vi "run_autoWC_v0.007.vi"(7 "long?":bool=TRUE, 8 "error in":errorcluster, 9 "HEK/slice options":enum16{"slice", "HEK"}(ring), 10 "auto run?":bool=TRUE, 11 "data in":T3={"daq_ao 1"="Dev1/ao0", "daq_ai 1"="Dev1/ai0", "experiment day folder"=path "C:/Users/sftlab/Documents/patcherBot_exp/data/test.lvm", "Multiclamp init error"=0, "Multiclamp Handle Out"=0, "sampling rate (Hz)"=20000, "trial name"=""}) -> (0 "error out":errorcluster)   [LabVIEW 2015]
uses:
  controls/Load and Save Controls_LV2009.llb/RWC_Actions.ctl
  wc_protocol_v1.003 Folder/whole_cell_protocol/Controls/clamp_profile.ctl
  controls/memtest_def.ctl
  Controls/Data.ctl
  wc_protocol_v1.003 Folder/whole_cell_protocol/Controls/cell_stats-v02.ctl
panel:
  out "HEK/slice options string":string
  out "config file":path=path "C:/multiBot/patcherBot/autoWCconfigs/autoWC_config_neuron-v07.ini"
  in  "load":bool
  in  "texts":enum32{"status", "comments", "release notes"}(tab)
  out "status":string
  in  "trial comments":string
  in  "release notes":string
  out "cell stats":T1 {"STD" format="%010.2f"; "Variance" format="%010.2f"; "Rt (MOhms)" format="%010.2f"; "tau (ms)" format="%08.2g"; "Cm (pF)" format="%08.2f"; "Ra (MOhms)" format="%010.2f"; "Rm (MOhms)" format="%010.2f"; "Ihold (pA)" format="%010.2f"}
  in  "save":bool
  in  "stop":bool
  in  "output":enum32{"VClamp", "IClamp"}(tab)
  out "Recorded currents (pA)":waveform(dbl)[](graph)
  out "Command steps (mV)":waveform(dbl)[](graph)
  out "Command steps (pA)":waveform(dbl)[](graph)
  out "Recorded voltage (mV)":waveform(dbl)[](graph)
  in  "run":bool
  in  "save as...":bool
  in  "update plots":bool
  in  "protocol creation":T2(tab)
  in  "DEBUG?":bool
  in  "auto WC run trigger":bool
  in  "twitter?":bool
  in  "config for long protocol":path=path "C:/multiBot/patcherBot/autoWCconfigs/autoWC_config_cellAttached-v01.ini"
  in  "config for standard protocol":path=path "C:/multiBot/patcherBot/autoWCconfigs/autoWC_config_neuron-v07.ini"
  in  "starting set":enum32{"Iprot", "Vprot", "Imemtest", "Vmemtest"}(tab)
  out "starting iprot cmd":waveform(dbl)[](graph)
  in  "Starting Iprot":T5={"Iclamp in"={"aLevel"=0.0, "aDelta"=0.0, "aDuration"=4000, "bLevel"=-200.0, "bDelta"=100.0, "bDuration"=4000, "cLevel"=0.0, "cDelta"=0.0, "cDuration"=4000}, "# iter"=6, "# reps IC"=1}
  out "starting vprot cmd":waveform(dbl)[](graph)
  in  "Starting Vprot":T6={"Vclamp in"={"aLevel"=0.0, "aDelta"=0.0, "aDuration"=40000, "bLevel"=-30.0, "bDelta"=10.0, "bDuration"=40000, "cLevel"=0.0, "cDelta"=0.0, "cDuration"=40000}, "# iter"=8, "# reps VC"=1}
  out "starting imemtest view":waveform(dbl)(graph)
  in  "Starting Iclamp memtest":T7={"Samples to Read"=2000, "Rate (Hz)"=20000.0, "Amplitude (mV/pA)"=-50.0, "Offset (mV/pA)"=0.0, "Frequency (Hz)"=10.0, "duty cycle (%)"=50.0, "phase"=0.0} {"phase" format="%.2p"; "duty cycle (%)" format="%0.2f"}
  out "starting vmemtest view":waveform(dbl)(graph)
  in  "Starting Vclamp memtest":T7={"Samples to Read"=2000, "Rate (Hz)"=20000.0, "Amplitude (mV/pA)"=10.0, "Offset (mV/pA)"=0.0, "Frequency (Hz)"=10.0, "duty cycle (%)"=50.0, "phase"=-90.0} {"phase" format="%.2p"; "duty cycle (%)" format="%0.2f"}
  in  "wait after init (s)":dbl
  in  "Starting sets":T8
  in  "wait after Starting set (s)":dbl
  in  "wait after Repeating set (s)":dbl
  in  "# sets":i32=18
  in  "Repeating sets":T8
  in  "repeating set":enum32{"Iprot", "Vprot", "Imemtest", "Vmemtest"}(tab)
  out "repeating iprot cmd":waveform(dbl)[](graph)
  in  "Repeating Iprot":T5={"Iclamp in"={"aLevel"=0.0, "aDelta"=0.0, "aDuration"=4000, "bLevel"=-200.0, "bDelta"=100.0, "bDuration"=4000, "cLevel"=0.0, "cDelta"=0.0, "cDuration"=4000}, "# iter"=6, "# reps IC"=1}
  out "repeating vprot cmd":waveform(dbl)[](graph)
  in  "Repeating Vprot":T6={"Vclamp in"={"aLevel"=0.0, "aDelta"=0.0, "aDuration"=40000, "bLevel"=-30.0, "bDelta"=10.0, "bDuration"=40000, "cLevel"=0.0, "cDelta"=0.0, "cDuration"=40000}, "# iter"=8, "# reps VC"=1}
  out "repeating imemtest cmd":waveform(dbl)(graph)
  in  "Repeating Iclamp memtest":T7={"Samples to Read"=2000, "Rate (Hz)"=20000.0, "Amplitude (mV/pA)"=-50.0, "Offset (mV/pA)"=0.0, "Frequency (Hz)"=10.0, "duty cycle (%)"=50.0, "phase"=0.0} {"phase" format="%.2p"; "duty cycle (%)" format="%0.2f"}
  out "repeating vmemtest cmd":waveform(dbl)(graph)
  in  "Repeating Vclamp memtest":T7={"Samples to Read"=2000, "Rate (Hz)"=20000.0, "Amplitude (mV/pA)"=10.0, "Offset (mV/pA)"=0.0, "Frequency (Hz)"=10.0, "duty cycle (%)"=50.0, "phase"=-90.0} {"phase" format="%.2p"; "duty cycle (%)" format="%0.2f"}
  in  "wait between protocols (s)":dbl
  in  "wait between sets (s)":dbl
  in  "ending set":enum32{"Iprot", "Vprot", "Imemtest", "Vmemtest"}(tab)
  out "ending iprot cmd":waveform(dbl)[](graph)
  in  "Ending Iprot":T5={"Iclamp in"={"aLevel"=0.0, "aDelta"=0.0, "aDuration"=4000, "bLevel"=-200.0, "bDelta"=100.0, "bDuration"=4000, "cLevel"=0.0, "cDelta"=0.0, "cDuration"=4000}, "# iter"=6, "# reps IC"=1}
  out "ending vprot cmd":waveform(dbl)[](graph)
  in  "Ending Vprot":T6={"Vclamp in"={"aLevel"=0.0, "aDelta"=0.0, "aDuration"=40000, "bLevel"=-30.0, "bDelta"=10.0, "bDuration"=40000, "cLevel"=0.0, "cDelta"=0.0, "cDuration"=40000}, "# iter"=8, "# reps VC"=1}
  out "ending imemtest cmd":waveform(dbl)(graph)
  in  "Ending Iclamp memtest":T7={"Samples to Read"=2000, "Rate (Hz)"=20000.0, "Amplitude (mV/pA)"=-50.0, "Offset (mV/pA)"=0.0, "Frequency (Hz)"=10.0, "duty cycle (%)"=50.0, "phase"=0.0} {"phase" format="%.2p"; "duty cycle (%)" format="%0.2f"}
  out "ending vmemtest cmd":waveform(dbl)(graph)
  in  "Ending Vclamp memtest":T7={"Samples to Read"=2000, "Rate (Hz)"=20000.0, "Amplitude (mV/pA)"=10.0, "Offset (mV/pA)"=0.0, "Frequency (Hz)"=10.0, "duty cycle (%)"=50.0, "phase"=-90.0} {"phase" format="%.2p"; "duty cycle (%)" format="%0.2f"}
  in  "Ending sets":T8
  in  "holding memtest":bool
  in  "holding set":enum32{"VClamp", "IClamp"}(tab)
  out "holding vmemtest cmd":waveform(dbl)(graph)
  in  "holding Vclamp memtest":T7={"Samples to Read"=2000, "Rate (Hz)"=20000.0, "Amplitude (mV/pA)"=10.0, "Offset (mV/pA)"=0.0, "Frequency (Hz)"=10.0, "duty cycle (%)"=50.0, "phase"=0.0} {"phase" format="%.2p"; "duty cycle (%)" format="%0.2f"}
  out "holding imemtest cmd":waveform(dbl)(graph)
  in  "holding Iclamp memtest":T7={"Samples to Read"=2000, "Rate (Hz)"=20000.0, "Amplitude (mV/pA)"=-50.0, "Offset (mV/pA)"=0.0, "Frequency (Hz)"=10.0, "duty cycle (%)"=50.0, "phase"=0.0} {"phase" format="%.2p"; "duty cycle (%)" format="%0.2f"}
  # "IClamp step protocol"
  # "x"
  # "VClamp step protocol"
  # "x"
  # "IClamp step protocol"
  # "x"
  # "VClamp step protocol"
  # "x"
  # "IClamp step protocol"
  # "x"
  # "VClamp step protocol"
  # "x"
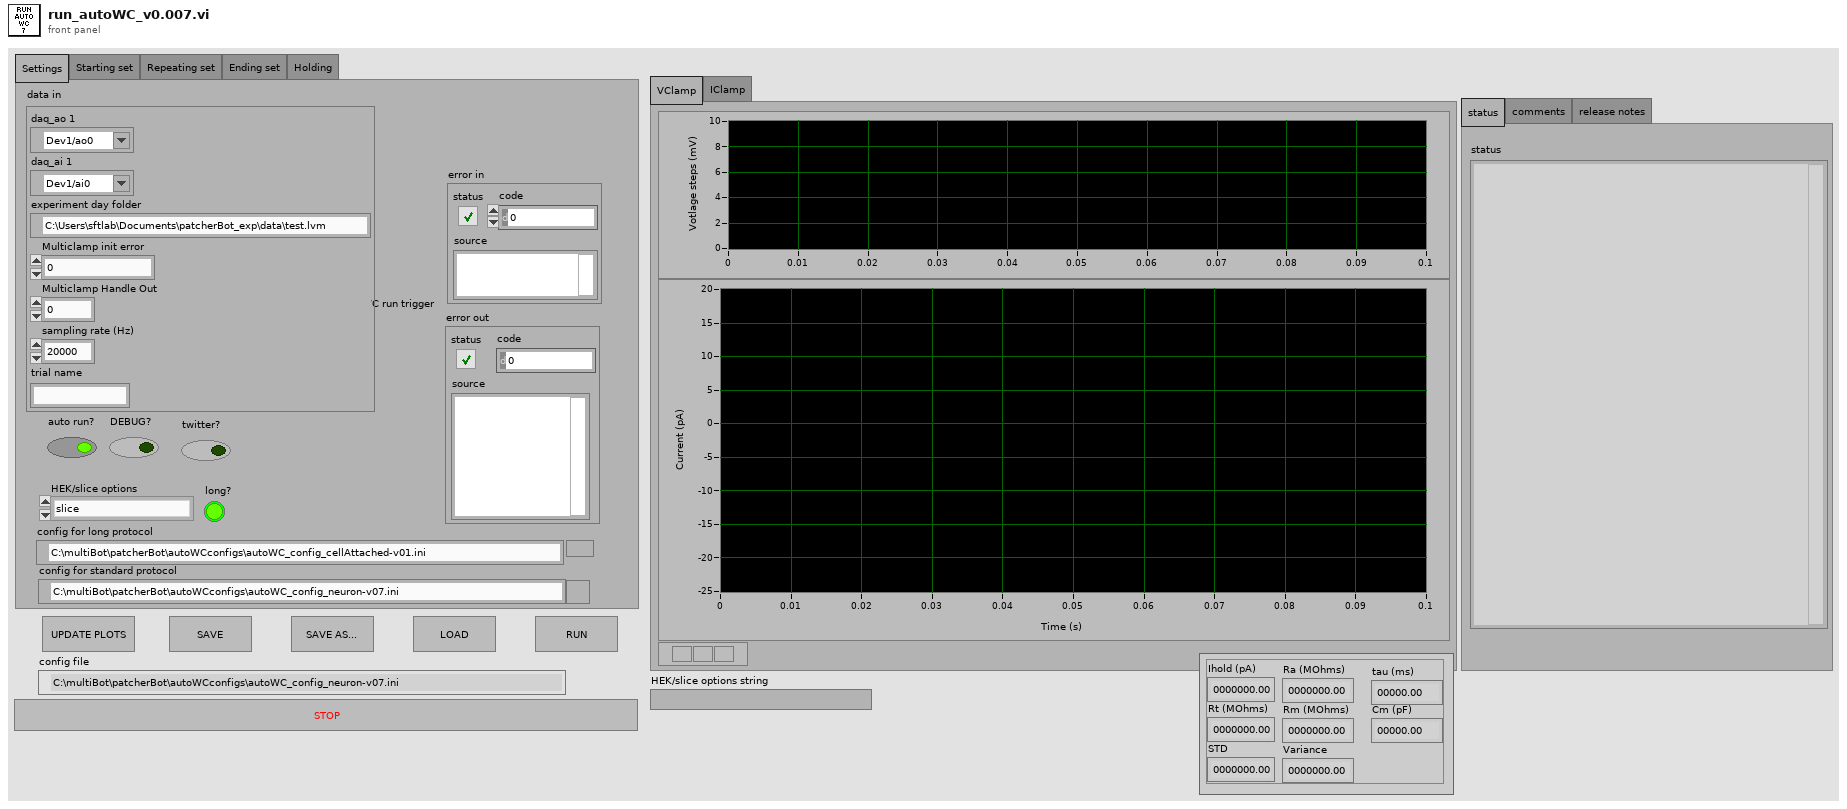
[diagram p1: front panel]
types:
  T1 = typedef "cell_stats-v02.ctl" = cluster{"Ihold (pA)":dbl, "Rm (MOhms)":dbl, "Ra (MOhms)":dbl, "Cm (pF)":dbl, "tau (ms)":dbl, "Rt (MOhms)":dbl, "Variance":dbl, "STD":dbl}
  T2 = enum32{"Settings", "Starting set", "Repeating set", "Ending set", "Holding"}
  T3 = typedef "Data.ctl" = cluster{"daq_ao 1":tag, "daq_ai 1":tag, "experiment day folder":path, "Multiclamp init error":i32, "Multiclamp Handle Out":u32, "sampling rate (Hz)":i32, "trial name":string}
  T4 = typedef "clamp_profile.ctl" = cluster{"aLevel":dbl, "aDelta":dbl, "aDuration":i32, "bLevel":dbl, "bDelta":dbl, "bDuration":i32, "cLevel":dbl, "cDelta":dbl, "cDuration":i32}
  T5 = cluster{"Iclamp in":T4, "# iter":i32, "# reps IC":i32}
  T6 = cluster{"Vclamp in":T4, "# iter":i32, "# reps VC":i32}
  T7 = typedef "memtest_def.ctl" = cluster{"Samples to Read":i32, "Rate (Hz)":dbl, "Amplitude (mV/pA)":dbl, "Offset (mV/pA)":dbl, "Frequency (Hz)":dbl, "duty cycle (%)":dbl, "phase":dbl}
  T8 = cluster{" Iprot":bool, " Vprot":bool, " Imemtest":bool, " Vmemtest":bool}
  T9 = typedef "RWC_Actions.ctl" = enum16{"Read", "Write", "Read and Create"}
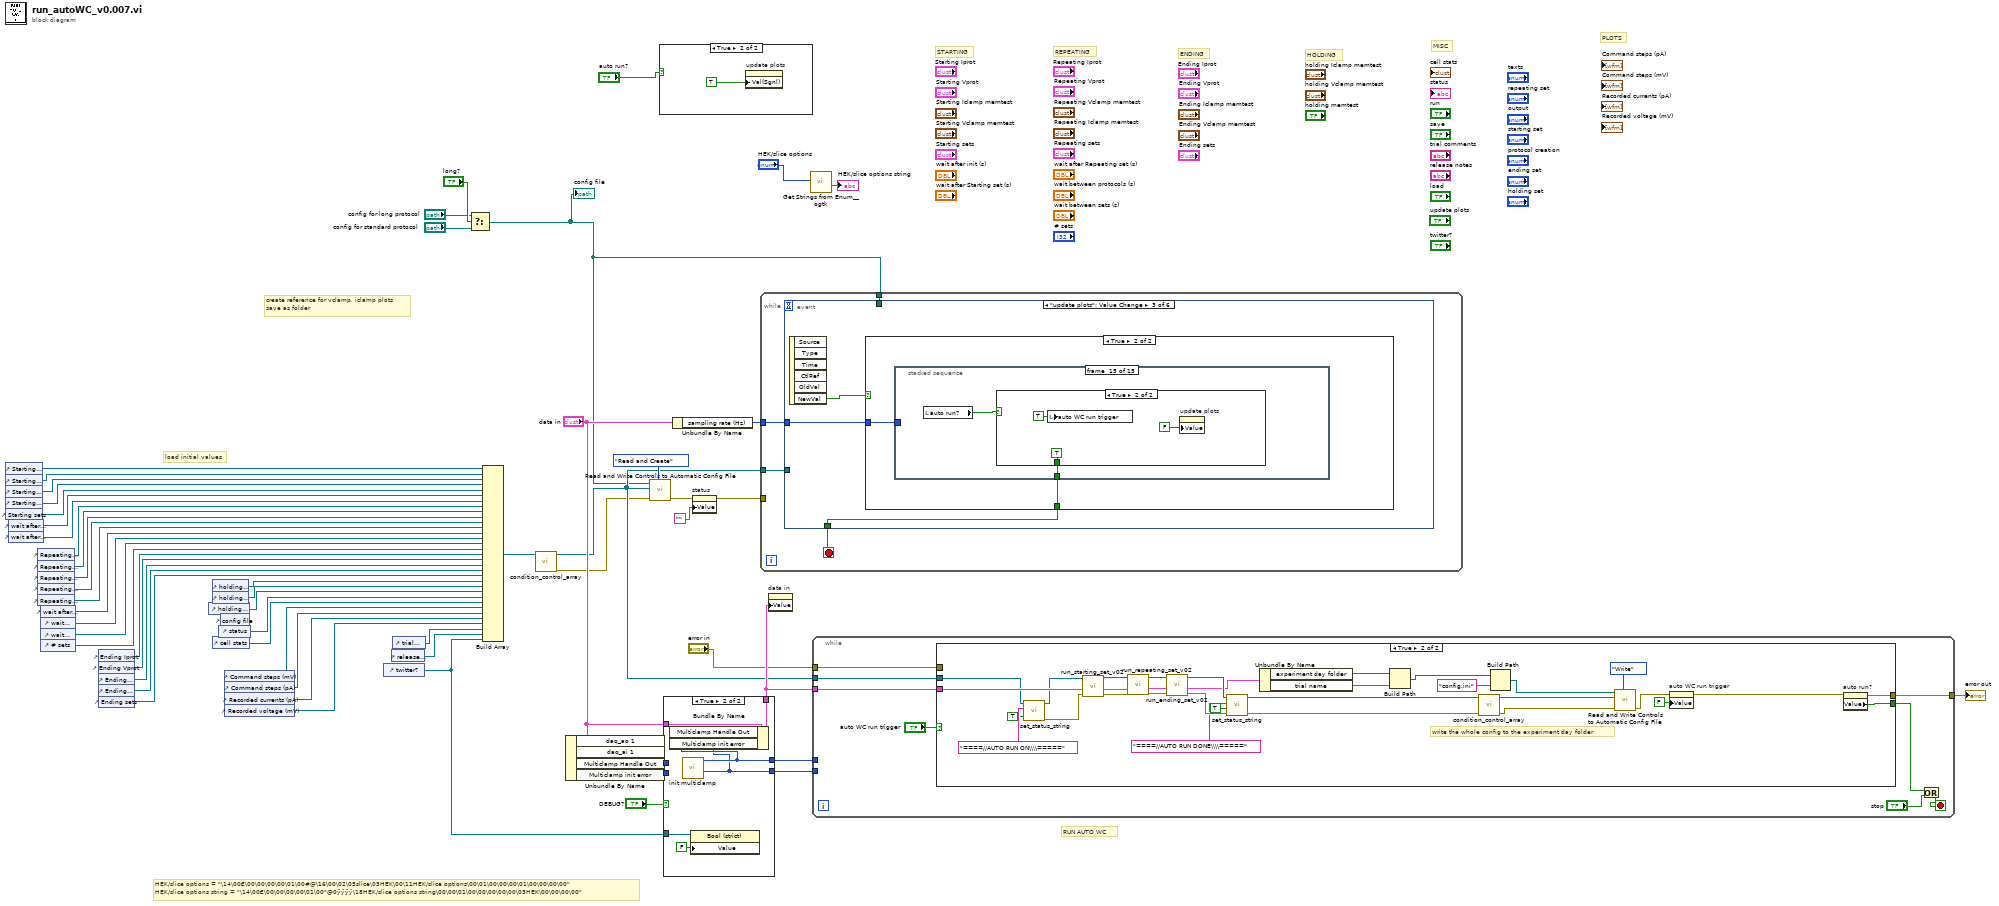
[diagram p0: block diagram]
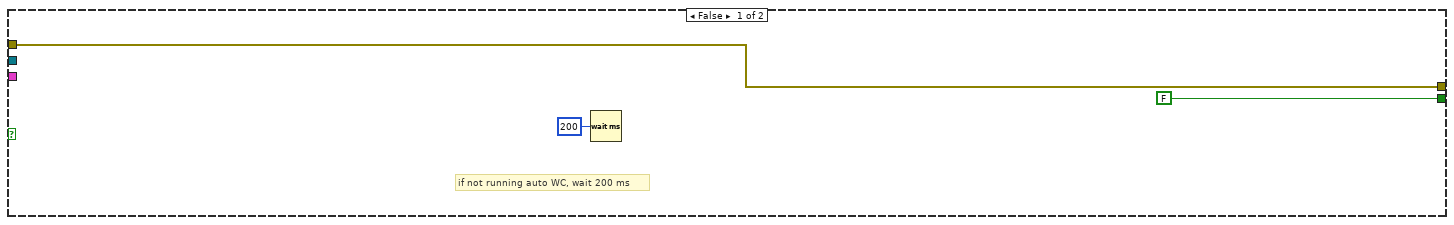
[diagram p4: hidden frame]
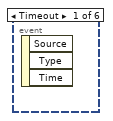
[diagram p5: hidden frame]
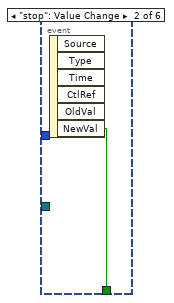
[diagram p6: hidden frame]
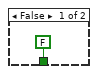
[diagram p7: hidden frame]
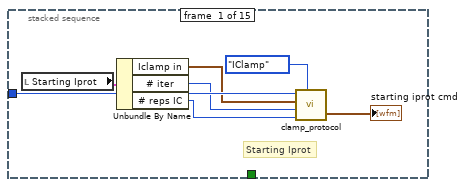
[diagram p8: hidden frame]
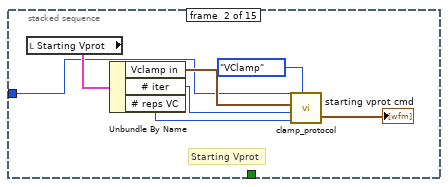
[diagram p9: hidden frame]
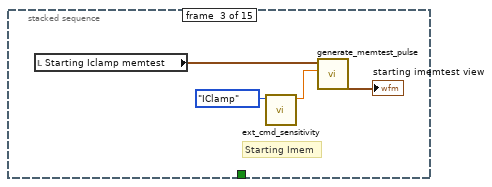
[diagram p10: hidden frame]
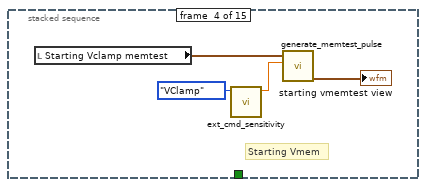
[diagram p11: hidden frame]
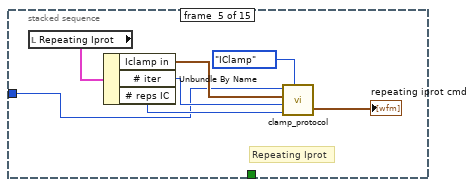
[diagram p12: hidden frame]
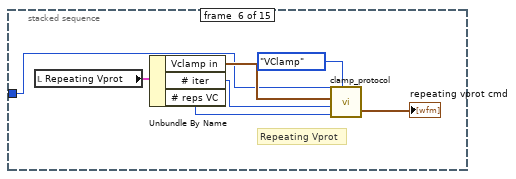
[diagram p13: hidden frame]
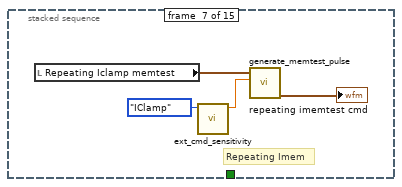
[diagram p14: hidden frame]
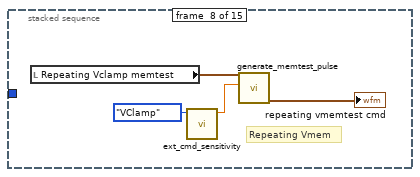
[diagram p15: hidden frame]
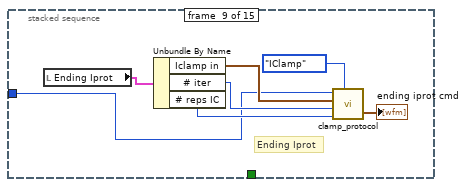
[diagram p16: hidden frame]
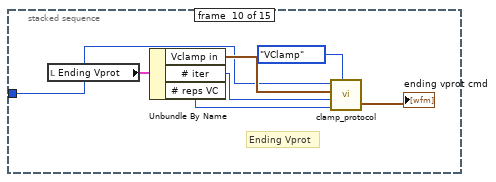
[diagram p17: hidden frame]
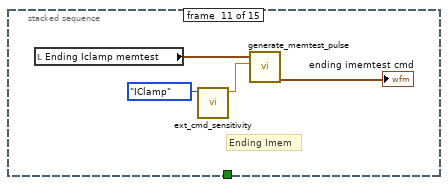
[diagram p18: hidden frame]
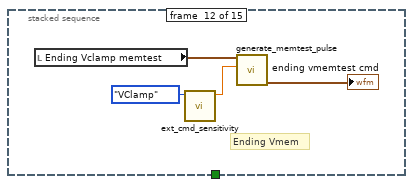
[diagram p19: hidden frame]
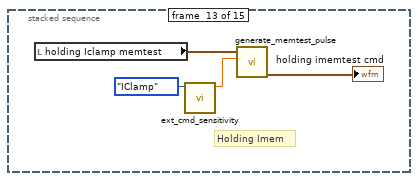
[diagram p20: hidden frame]
diagram:
  # "HEK/slice options = \"\\14\\00€\\00\\00\\00\\00\\01\\00#@\\16\\00\\02\\05slice\\03HEK\\00\\11HEK/slice options\\00\\01\\00\\00\\00\\01\\00\\00\\00\\00\"\nHEK/slice options string = \"\\14\\00€\\00\\00\\00\\00\\01\\00\"@0ÿÿÿÿ\\18HEK/slice options string\\00\\00\\01\\00\\00\\00\\00\\00\\03HEK\\00\\00\\00\\00\""
  # "PLOTS"
  # "MISC"
  # "create reference for vclamp, iclamp plots\nsave as folder"
  # "load initial values"
  # "HOLDING"
  # "ENDING"
  # "REPEATING"
  # "STARTING"
  # "RUN AUTO WC"
  n1 = control-ref of="Starting Iprot"() -> (w35:refnum<vi>)
  n2 = control-ref of="Starting Vprot"() -> (w34:refnum<vi>)
  n3 = control-ref of="Starting Iclamp memtest"() -> (w33:refnum<vi>)
  n4 = control-ref of="Starting Vclamp memtest"() -> (w32:refnum<vi>)
  n5 = control-ref of="Starting sets"() -> (w36:refnum<vi>)
  n6 = control-ref of="wait after init (s)"() -> (w37:refnum<vi>)
  n7 = control-ref of="wait after Starting set (s)"() -> (w38:refnum<vi>)
  n8 = control-ref of="Repeating Iprot"() -> (w39:refnum<vi>)
  n9 = control-ref of="Repeating Vprot"() -> (w40:refnum<vi>)
  n10 = control-ref of="Repeating Vclamp memtest"() -> (w41:refnum<vi>)
  n11 = control-ref of="Repeating Iclamp memtest"() -> (w42:refnum<vi>)
  n12 = control-ref of="Repeating sets"() -> (w43:refnum<vi>)
  n13 = control-ref of="wait after Repeating set (s)"() -> (w44:refnum<vi>)
  n14 = control-ref of="wait between protocols (s)"() -> (w45:refnum<vi>)
  n15 = control-ref of="wait between sets (s)"() -> (w46:refnum<vi>)
  n16 = control-ref of="# sets"() -> (w47:refnum<vi>)
  n17 = control-ref of="Ending Iprot"() -> (w48:refnum<vi>)
  n18 = control-ref of="Ending Vprot"() -> (w49:refnum<vi>)
  n19 = control-ref of="Ending Iclamp memtest"() -> (w50:refnum<vi>)
  n20 = control-ref of="Ending Vclamp memtest"() -> (w51:refnum<vi>)
  n21 = control-ref of="Ending sets"() -> (w52:refnum<vi>)
  n22 = control-ref of="holding memtest"() -> (w55:refnum<vi>)
  n23 = control-ref of="holding Iclamp memtest"() -> (w53:refnum<vi>)
  n24 = control-ref of="holding Vclamp memtest"() -> (w54:refnum<vi>)
  n25 = control-ref of="cell stats"() -> (w26:refnum<vi>)
  n26 = control-ref of="status"() -> (w27:refnum<vi>)
  n27 = control-ref of="config file"() -> ()  [unwired: 1 out]
  n28 = control-ref of="Command steps (mV)"() -> (w14:refnum<vi>)
  n29 = control-ref of="Command steps (pA)"() -> (w13:refnum<vi>)
  n30 = control-ref of="Recorded currents (pA)"() -> (w12:refnum<vi>)
  n31 = control-ref of="Recorded voltage (mV)"() -> (w11:refnum<vi>)
  n32 = control-ref of="twitter?"() -> (w7:refnum<vi>)
  n33 = control-ref of="release notes"() -> (w15:refnum<vi>)
  n34 = control-ref of="trial comments"() -> (w16:refnum<vi>)
  n35 = Select(t="config for long protocol", s="long?", f="config for standard protocol") -> (s? t:f=w1:path)
  "config file" <- w1
  n36 = Build Array(w35, w34, w33, w32, w36, w37, w38, w39, w40, w41, w42, w43, w44, w45, w46, w47, w48, w49, w50, w51, w52, w53, w54, w55, w27, w26, w14, w13, w12, w11, w16, w15, w7) -> (w10:refnum<vi>[])
  n37 = call "condition_control_array.vi"("control array in"=w10) -> ("error out"=w8:errorcluster, "control array out"=w9:refnum<vi>[])  [unwired: 9 in]
  n38 = Unbundle By Name("data in") -> ("Multiclamp Handle Out"=w25:u32, "Multiclamp init error"=w24:i32)  [unwired: 2 out]
  n39 = call "Read and Write Controls to Automatic Config File.vi"("Action"=RWC_Actions."Read and Create", "error in"=w8, "Control References"=w9, "filepath"=w1) -> ("error out"=w23:errorcluster)  [unwired: 7 in]
  n40 = case shown="True" "auto run?" {
    frame False {
    }
    frame True {
      n41 = property on="update plots" class="Bool (strict)"("Val(Sgnl)"=TRUE ("update plots")) -> ()  [unwired: 2 in, 2 out]
    }
  }
  n42 = case shown="True" "DEBUG?" {
    tunnel: [w61 w67] -> w29
    tunnel: [w60 w66] -> w28
    tunnel: w25 -> [w61 _]
    tunnel: w24 -> [w60 _]
    tunnel: "data in" -> [w59 w65]
    tunnel: [w59 w64] -> w19
    tunnel: w7 -> [_ w63]
    frame False {
    }
    frame True {
      n43 = call "init multiclamp.vi"() -> ("Error out"=w66:i32, "Multiclamp Handle Out"=w67:u32)  [unwired: 9 in, 1 out]
      n44 = Bundle By Name(cluster=w65, "Multiclamp Handle Out"=w67, "Multiclamp init error"=w66) -> (w64:T3)
      n45 = property class="Bool (strict)"(reference=w63, "Value"=FALSE) -> ()  [unwired: 1 in, 2 out]
    }
  }
  n46 = Unbundle By Name("data in") -> ("sampling rate (Hz)"=w56:i32)
  n47 = property on="status" class="Str"(error in=w23, "Value"="") -> (error out=w22:errorcluster)  [unwired: 1 in, 1 out]
  n48 = while {
    tunnel: w56 -> [w70]
    tunnel: w1 -> [w69]
    tunnel: w22 -> [_]
    tunnel: w9 -> [w68]
    stop <- w71 stop-if-true
    n49 = event shown="[2] \"update plots\": Value Change" {
      selector: _ -> [_ _ _ _ _ _]
      dyn-events: _ -> [_ _ _ _ _ _]
      timeout: _ -> [_ _ _ _ _ _]
      tunnel: [_ w72 w73 _ _ _] -> w71
      tunnel: w70 -> [_ _ w74 _ _ _]
      tunnel: w69 -> [_ _ _ _ w163 _]
      tunnel: w68 -> [_ _ _ _ w162 w179]
      event Timeout {
        n50 = event-data() -> ()  [unwired: 1 in, 3 out]
      }
      event "stop": Value Change {
        n51 = event-data() -> ("NewVal"=w72:bool)  [unwired: 1 in, 5 out]
      }
      event "update plots": Value Change {
        n52 = event-data() -> ("NewVal"=w75:bool)  [unwired: 1 in, 5 out]
        n53 = case shown="True" w75 {
          tunnel: w74 -> [_ w78]
          tunnel: [FALSE w77] -> w73
          frame False {
          }
          frame True {
            n54 = stacked-sequence {
              tunnel: w78 -> [w85 w86 _ _ w103 w109 _ _ w123 w131 _ _ _ _ _]
              tunnel: [_ _ _ _ _ _ _ _ _ _ _ _ _ _ w153] -> w77
              frame #0 {
                # "Starting Iprot"
                n55 = local read "Starting Iprot"() -> (w83:T5)
                n56 = Unbundle By Name(w83) -> ("Iclamp in"=w82:T4, "# iter"=w81:i32, "# reps IC"=w80:i32)
                n57 = call "clamp_protocol.vi"("which clamp"=enum16{"VClamp", "IClamp"}."IClamp", "# reps"=w80, "# Iterations"=w81, "clamp in"=w82, "sampling rate (Hz)"=w85) -> ("View profile (wvfrms)"=→"starting iprot cmd":waveform(dbl)[])  [unwired: 2 out]
              }
              frame #1 {
                # "Starting Vprot"
                n58 = local read "Starting Vprot"() -> (w90:T6)
                n59 = Unbundle By Name(w90) -> ("Vclamp in"=w91:T4, "# iter"=w88:i32, "# reps VC"=w87:i32)
                n60 = call "clamp_protocol.vi"("which clamp"=enum16{"VClamp", "IClamp"}."VClamp", "# reps"=w87, "# Iterations"=w88, "clamp in"=w91, "sampling rate (Hz)"=w86) -> ("View profile (wvfrms)"=→"starting vprot cmd":waveform(dbl)[])  [unwired: 2 out]
              }
              frame #2 {
                # "Starting Imem"
                n61 = local read "Starting Iclamp memtest"() -> (w93:T7)
                n62 = call "ext_cmd_sensitivity.vi"("which clamp"=enum16{"VClamp", "IClamp"}."IClamp") -> ("division factor"=w96:dbl)  [unwired: 10 in]
                n63 = call "generate_memtest_pulse.vi"("external cmd sensitivity"=w96, "memtest"=w93) -> ("view memtest"=→"starting imemtest view":waveform(dbl))  [unwired: 8 in, 1 out]
              }
              frame #3 {
                # "Starting Vmem"
                n64 = local read "Starting Vclamp memtest"() -> (w97:T7)
                n65 = call "ext_cmd_sensitivity.vi"("which clamp"=enum16{"VClamp", "IClamp"}."VClamp") -> ("division factor"=w100:dbl)  [unwired: 10 in]
                n66 = call "generate_memtest_pulse.vi"("external cmd sensitivity"=w100, "memtest"=w97) -> ("view memtest"=→"starting vmemtest view":waveform(dbl))  [unwired: 8 in, 1 out]
              }
              frame #4 {
                # "Repeating Iprot"
                n67 = local read "Repeating Iprot"() -> (w101:T5)
                n68 = Unbundle By Name(w101) -> ("Iclamp in"=w106:T4, "# iter"=w105:i32, "# reps IC"=w104:i32)
                n69 = call "clamp_protocol.vi"("which clamp"=enum16{"VClamp", "IClamp"}."IClamp", "# reps"=w104, "# Iterations"=w105, "clamp in"=w106, "sampling rate (Hz)"=w103) -> ("View profile (wvfrms)"=→"repeating iprot cmd":waveform(dbl)[])  [unwired: 2 out]
              }
              frame #5 {
                # "Repeating Vprot"
                n70 = local read "Repeating Vprot"() -> (w108:T6)
                n71 = Unbundle By Name(w108) -> ("Vclamp in"=w113:T4, "# iter"=w112:i32, "# reps VC"=w111:i32)
                n72 = call "clamp_protocol.vi"("which clamp"=enum16{"VClamp", "IClamp"}."VClamp", "# reps"=w111, "# Iterations"=w112, "clamp in"=w113, "sampling rate (Hz)"=w109) -> ("View profile (wvfrms)"=→"repeating vprot cmd":waveform(dbl)[])  [unwired: 2 out]
              }
              frame #6 {
                # "Repeating Imem"
                n73 = local read "Repeating Iclamp memtest"() -> (w115:T7)
                n74 = call "ext_cmd_sensitivity.vi"("which clamp"=enum16{"VClamp", "IClamp"}."IClamp") -> ("division factor"=w118:dbl)  [unwired: 10 in]
                n75 = call "generate_memtest_pulse.vi"("external cmd sensitivity"=w118, "memtest"=w115) -> ("view memtest"=→"repeating imemtest cmd":waveform(dbl))  [unwired: 8 in, 1 out]
              }
              frame #7 {
                # "Repeating Vmem"
                n76 = local read "Repeating Vclamp memtest"() -> (w119:T7)
                n77 = call "ext_cmd_sensitivity.vi"("which clamp"=enum16{"VClamp", "IClamp"}."VClamp") -> ("division factor"=w122:dbl)  [unwired: 10 in]
                n78 = call "generate_memtest_pulse.vi"("external cmd sensitivity"=w122, "memtest"=w119) -> ("view memtest"=→"repeating vmemtest cmd":waveform(dbl))  [unwired: 8 in, 1 out]
              }
              frame #8 {
                # "Ending Iprot"
                n79 = local read "Ending Iprot"() -> (w124:T5)
                n80 = Unbundle By Name(w124) -> ("Iclamp in"=w128:T4, "# iter"=w127:i32, "# reps IC"=w126:i32)
                n81 = call "clamp_protocol.vi"("which clamp"=enum16{"VClamp", "IClamp"}."IClamp", "# reps"=w126, "# Iterations"=w127, "clamp in"=w128, "sampling rate (Hz)"=w123) -> ("View profile (wvfrms)"=→"ending iprot cmd":waveform(dbl)[])  [unwired: 2 out]
              }
              frame #9 {
                # "Ending Vprot"
                n82 = local read "Ending Vprot"() -> (w130:T6)
                n83 = Unbundle By Name(w130) -> ("Vclamp in"=w135:T4, "# iter"=w134:i32, "# reps VC"=w133:i32)
                n84 = call "clamp_protocol.vi"("which clamp"=enum16{"VClamp", "IClamp"}."VClamp", "# reps"=w133, "# Iterations"=w134, "clamp in"=w135, "sampling rate (Hz)"=w131) -> ("View profile (wvfrms)"=→"ending vprot cmd":waveform(dbl)[])  [unwired: 2 out]
              }
              frame #10 {
                # "Ending Imem"
                n85 = local read "Ending Iclamp memtest"() -> (w137:T7)
                n86 = call "ext_cmd_sensitivity.vi"("which clamp"=enum16{"VClamp", "IClamp"}."IClamp") -> ("division factor"=w140:dbl)  [unwired: 10 in]
                n87 = call "generate_memtest_pulse.vi"("external cmd sensitivity"=w140, "memtest"=w137) -> ("view memtest"=→"ending imemtest cmd":waveform(dbl))  [unwired: 8 in, 1 out]
              }
              frame #11 {
                # "Ending Vmem"
                n88 = local read "Ending Vclamp memtest"() -> (w141:T7)
                n89 = call "ext_cmd_sensitivity.vi"("which clamp"=enum16{"VClamp", "IClamp"}."VClamp") -> ("division factor"=w144:dbl)  [unwired: 10 in]
                n90 = call "generate_memtest_pulse.vi"("external cmd sensitivity"=w144, "memtest"=w141) -> ("view memtest"=→"ending vmemtest cmd":waveform(dbl))  [unwired: 8 in, 1 out]
              }
              frame #12 {
                # "Holding Imem"
                n91 = local read "holding Iclamp memtest"() -> (w145:T7)
                n92 = call "ext_cmd_sensitivity.vi"("which clamp"=enum16{"VClamp", "IClamp"}."IClamp") -> ("division factor"=w148:dbl)  [unwired: 10 in]
                n93 = call "generate_memtest_pulse.vi"("external cmd sensitivity"=w148, "memtest"=w145) -> ("view memtest"=→"holding imemtest cmd":waveform(dbl))  [unwired: 8 in, 1 out]
              }
              frame #13 {
                # "Holding Vmem"
                n94 = local read "holding Vclamp memtest"() -> (w149:T7)
                n95 = call "ext_cmd_sensitivity.vi"("which clamp"=enum16{"VClamp", "IClamp"}."VClamp") -> ("division factor"=w152:dbl)  [unwired: 10 in]
                n96 = call "generate_memtest_pulse.vi"("external cmd sensitivity"=w152, "memtest"=w149) -> ("view memtest"=→"holding vmemtest cmd":waveform(dbl))  [unwired: 8 in, 1 out]
              }
              frame #14 {
                n97 = local read "auto run?"() -> (w154:bool)
                n98 = case shown="True" w154 {
                  tunnel: [FALSE TRUE] -> w153
                  frame False {
                  }
                  frame True {
                    n99 = local write "auto WC run trigger"(TRUE ("auto WC run trigger")) -> ()
                    n100 = property on="update plots" class="Bool (strict)"("Value"=FALSE ("Value (Signaling)")) -> ()  [unwired: 2 in, 2 out]
                  }
                }
              }
            }
          }
        }
      }
      event "run": Value Change {
        n101 = event-data() -> ("NewVal"=w159:bool)  [unwired: 1 in, 5 out]
        n102 = case shown="True" w159 {
          selector: w159 -> [_ w160]
          frame False {
          }
          frame True {
            n103 = property on="auto WC run trigger" class="Bool (strict)"("Value"=w160) -> ()  [unwired: 2 in, 2 out]
          }
        }
      }
      event "save", "save as...": Value Change {
        n104 = event-data() -> ("NewVal"=w161:bool)  [unwired: 1 in, 5 out]
        n105 = case shown="True" w161 {
          tunnel: "save as..." -> [_ w169]
          tunnel: w163 -> [_ w168]
          tunnel: w162 -> [_ w167]
          frame False {
          }
          frame True {
            n106 = case shown="True" w169 {
              tunnel: w168 -> [w175 _]
              tunnel: [w175 w177] -> w166
              tunnel: [FALSE ("cancelled") w176] -> w165
              frame False {
              }
              frame True {
                n107 = call "select config"("prompt"="Save as...") -> ("selected path"=w177:path, "cancelled"=w176:bool)  [unwired: 11 in, 2 out]
                n108 = local write "config file"(w177) -> ()
              }
            }
            n109 = case shown="False" w165 {
              tunnel: w167 -> [w171 _]
              tunnel: w166 -> [w172 _]
              frame False {
                n110 = call "condition_control_array.vi"("control array in"=w171) -> ("control array out"=w170:refnum<vi>[])  [unwired: 9 in, 1 out]
                n111 = call "Read and Write Controls to Automatic Config File.vi"("Action"=RWC_Actions."Write", "Control References"=w170, "filepath"=w172) -> ()  [unwired: 8 in, 1 out]
              }
              frame True {
              }
            }
          }
        }
      }
      event "load": Value Change {
        n112 = event-data() -> ("NewVal"=w180:bool)  [unwired: 1 in, 5 out]
        n113 = case shown="True" w180 {
          tunnel: w179 -> [_ w183]
          frame False {
          }
          frame True {
            n114 = call "load config"() -> ("selected path"=w182:path, "cancelled"=w181:bool)  [unwired: 12 in, 2 out]
            n115 = case shown="False" w181 {
              tunnel: w183 -> [w186 _]
              tunnel: w182 -> [w184 _]
              frame False {
                n116 = call "Read and Write Controls to Automatic Config File.vi"("Action"=RWC_Actions."Read", "Control References"=w186, "filepath"=w184) -> ()  [unwired: 8 in, 1 out]
                n117 = local write "config file"(w184) -> ()
              }
              frame True {
              }
            }
          }
        }
      }
    }
  }
  n118 = property on="data in" class="Clust (strict)"("Value"=w19) -> ()  [unwired: 2 in, 2 out]
  n119 = call "Get Strings from Enum__ogtk.vi"("Enum"="HEK/slice options") -> ("String Value"=→"HEK/slice options string":string)  [unwired: 7 in, 3 out]
  n120 = while {
    tunnel: w29 -> [_]
    tunnel: w28 -> [_]
    tunnel: w9 -> [w193]
    tunnel: w19 -> [w192]
    tunnel: [w188] -> w18
    tunnel: "error in" -> [w187]
    stop <- w191 stop-if-true
    n121 = case shown="True" "auto WC run trigger" {
      tunnel: w193 -> [_ w227]
      tunnel: w192 -> [_ w228]
      tunnel: [FALSE ("Value") w222] -> w189
      tunnel: [w195 w205] -> w188
      tunnel: w187 -> [w195 _]
      frame False {
        # "if not running auto WC, wait 200 ms"
        n122 = Wait (ms)(milliseconds to wait=u32 200) -> ()  [unwired: 1 out]
      }
      frame True {
        # "write the whole config to the experiment day folder"
        n123 = call "set_status_string.vi"("new line?"=TRUE, "status string in"="====//AUTO RUN ON\\\\=====", "controls array"=w227) -> ("error out"=w219:errorcluster, "controls array out"=w226:refnum<vi>[])  [unwired: 7 in]
        n124 = call "run_starting_set_v02.vi"("error in"=w219, "data in"=w228, "controls array in"=w226) -> ("error out"=w218:errorcluster, "data out"=w220:T3, "control array out"=w221:refnum<vi>[])  [unwired: 6 in]
        n125 = call "run_repeating_set_v02.vi"("error in"=w218, "data in"=w220, "controls array in"=w221) -> ("error out"=w215:errorcluster, "data out"=w216:T3, "control array out"=w217:refnum<vi>[])  [unwired: 6 in]
        n126 = call "run_ending_set_v02.vi"("error in"=w215, "data in"=w216, "controls array in"=w217) -> ("error out"=w213:errorcluster, "data out"=w209:T3, "control array out"=w214:refnum<vi>[])  [unwired: 6 in]
        n127 = call "set_status_string.vi"("error in"=w213, "new line?"=TRUE, "status string in"="====//AUTO RUN DONE\\\\=====", "controls array"=w214) -> ("error out"=w199:errorcluster, "controls array out"=w201:refnum<vi>[])  [unwired: 6 in]
        n128 = Unbundle By Name(w209) -> ("experiment day folder"=w204:path, "trial name"=w203:string)
        n129 = Build Path(base path=w204, name or relative path=w203) -> (appended path=w202:path)
        n130 = call "condition_control_array.vi"("error in"=w199, "control array in"=w201) -> ("error out"=w198:errorcluster, "control array out"=w200:refnum<vi>[])  [unwired: 8 in]
        n131 = Build Path(base path=w202, name or relative path="config.ini") -> (appended path=w207:path)
        n132 = call "Read and Write Controls to Automatic Config File.vi"("Action"=RWC_Actions."Write", "error in"=w198, "Control References"=w200, "filepath"=w207) -> ("error out"=w206:errorcluster)  [unwired: 7 in]
        n133 = property on="auto WC run trigger" class="Bool (strict)"(error in=w206, "Value"=FALSE ("auto WC run trigger")) -> (error out=w223:errorcluster)  [unwired: 1 in, 1 out]
        n134 = property on="auto run?" class="Bool (strict)"(error in=w223) -> (error out=w205:errorcluster, "Value"=w222:bool)  [unwired: 1 in, 1 out]
      }
    }
    n135 = Or(x=w189, y="stop") -> (x .or. y?=w191:bool)
  }
  "error out" <- w18
